vi "General Enqueue Function - Data Logger.vi"   [LabVIEW 2014]
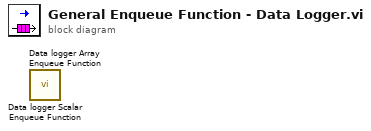
[diagram p0: block diagram]
diagram:
  n1 = call "Data logger Scalar Enqueue Function.vi"() -> ()  [unwired: 14 in, 2 out]
  n2 = call "Data logger Array Enqueue Function.vi"() -> ()  [unwired: 14 in, 2 out]
